vi "RLC Transfer Function Magnitude.vi"(0 "Start frequency, Hz":dbl, 1 "Circuit Type":T2, 5 "Stop frequency, Hz":dbl=10000.0, 7 "Step frequency, Hz":dbl=1.0 format="%#_13g", 11 "error in (no error)":errorcluster, 12 "R, Ohm":dbl=10.0 format="%#_13g", 13 "L, H":dbl=0.01 format="%#_13g", 14 "C, F":dbl=7.5e-06 format="%#_13g") -> (4 "RLC Circuit Transfer function (magnitude)":cluster{"X":dbl[], "Y":dbl[]}(graph), 6 "RLC Circuit Transfer function\n (magnitude) Image Data":T1, 8 "RLC Circuit Transfer function (magnitude) Picture":picture, 10 "JSON string":string, 15 "error out":errorcluster)   [LabVIEW 2019]
uses:
  Types/Circuit Type Enum.ctl
  <vilib>/picture/picture.llb/imagedata.ctl
  XY Graph Data Type.ctl
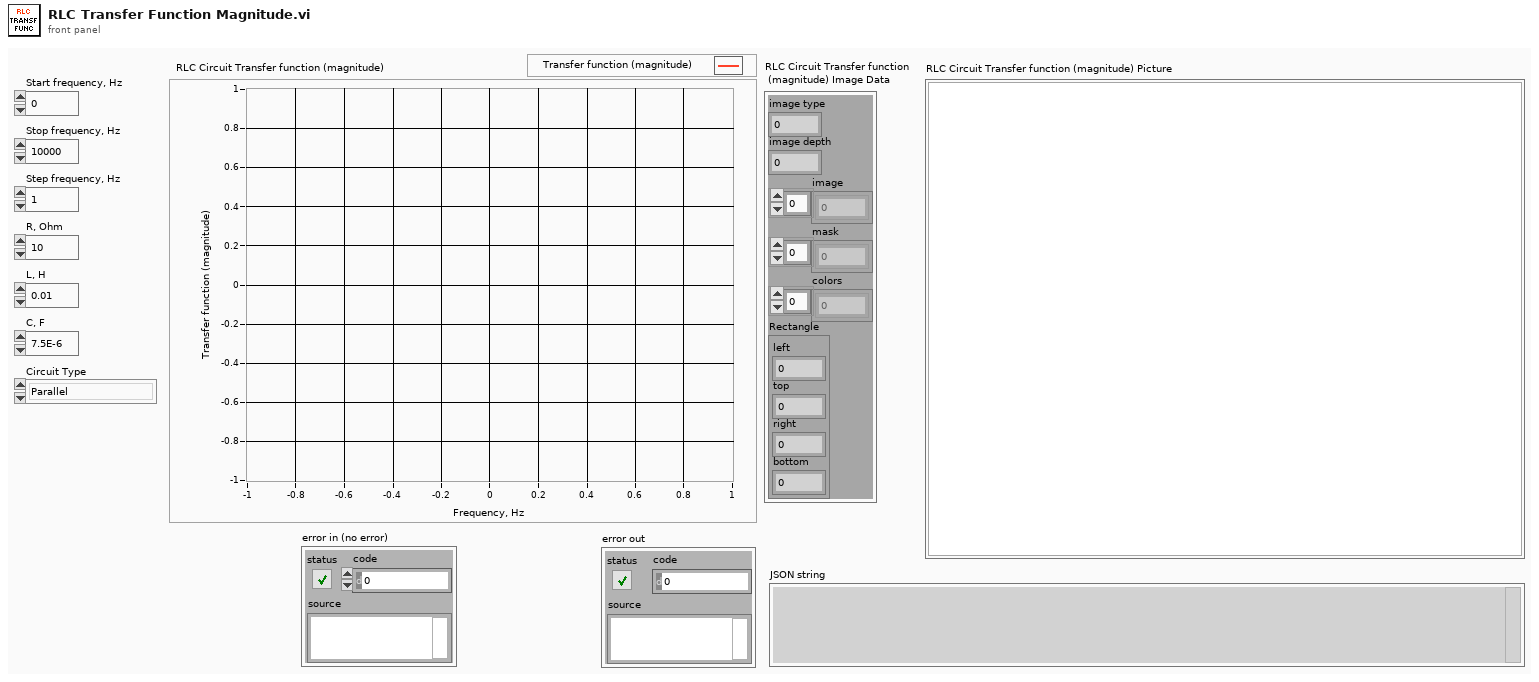
[diagram p1: front panel]
types:
  T1 = typedef "imagedata.ctl" = cluster{"image type":i32, "image depth":i32, "image":u8[], "mask":u8[], "colors":u32[], "Rectangle":cluster{"left":i16, "top":i16, "right":i16, "bottom":i16}}
  T2 = typedef "Circuit Type Enum.ctl" = enum16{"Parallel", "Serial"}
  T3 = typedef "XY Graph Data Type.ctl" = cluster{"X":dbl[], "Y":dbl[]}
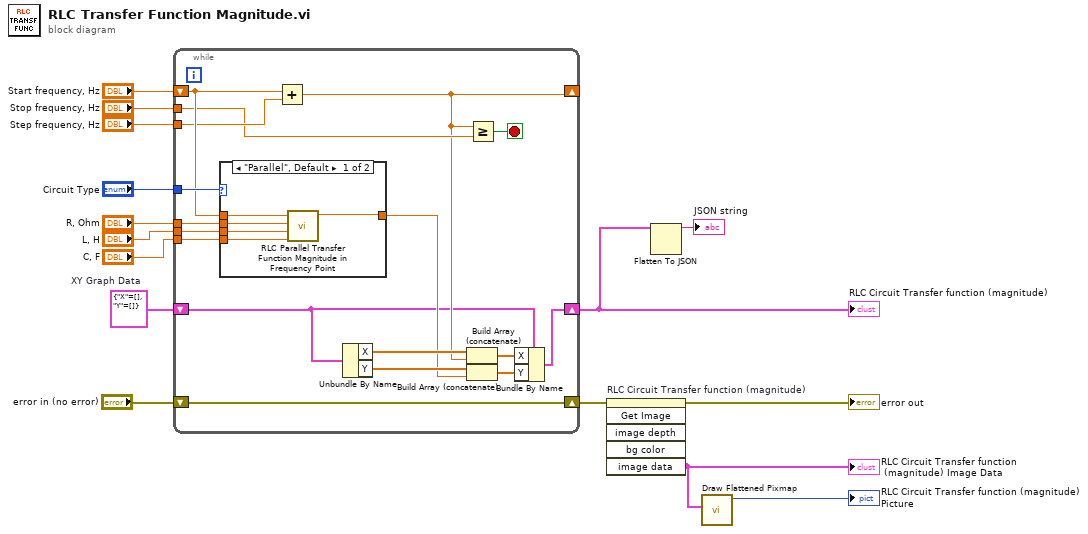
[diagram p0: block diagram]
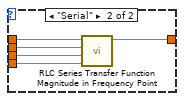
[diagram p2: hidden frame]
diagram:
  w3 = T3 {"X"=[], "Y"=[]}  # XY Graph Data
  n1 = while {
    tunnel: "R, Ohm" -> [w32]
    tunnel: "L, H" -> [w31]
    tunnel: "C, F" -> [w30]
    tunnel: "Circuit Type" -> [w29]
    tunnel: "Stop frequency, Hz" -> [w25]
    tunnel: "Step frequency, Hz" -> [w27]
    shift-right: [w21] -> _
    shift-left: "Start frequency, Hz" -> [w28]
    shift-right: [w16] -> w2
    shift-left: w3 -> [w19]
    shift-right: [w24] -> w7
    shift-left: "error in (no error)" -> [w24]
    stop <- w26 stop-if-true
    n2 = case shown="\"Parallel\", Default" w29 {
      tunnel: w32 -> [w36 w42]
      tunnel: w31 -> [w35 w41]
      tunnel: w30 -> [w34 w40]
      tunnel: w28 -> [w37 w39]
      tunnel: [w33 w38] -> w20
      frame "Parallel", Default {
        n3 = call "RLC Parallel Transfer Function Magnitude in Frequency Point.vi"("C, F"=w34, "L, H"=w35, "R, Ohm"=w36, "F, Hz"=w37) -> ("H(f)"=w33:dbl)  [unwired: 7 in]
      }
      frame "Serial" {
        n4 = call "RLC Series Transfer Function Magnitude in Frequency Point.vi"("C, F"=w40, "L, H"=w41, "R, Ohm"=w42, "F, Hz"=w39) -> ("H(f)"=w38:dbl)  [unwired: 7 in]
      }
    }
    n5 = Add(x=w28, y=w27) -> (x+y=w21:dbl)
    n6 = Unbundle By Name(w19) -> ("X"=w23:dbl[], "Y"=w22:dbl[])
    n7 = Build Array (concatenate)(w23, w21) -> (w18:dbl[])
    n8 = Build Array (concatenate)(w22, w20) -> (w17:dbl[])
    n9 = Greater Or Equal?(x=w21, y=w25) -> (x >= y?=w26:bool)
    n10 = Bundle By Name(cluster=w19, "X"=w18, "Y"=w17) -> (w16:T3)
  }
  "RLC Circuit Transfer function (magnitude)" <- w2
  n11 = invoke on="RLC Circuit Transfer function (magnitude)" class="XYGraph (strict)" method="Get Image"(error in=w7) -> (error out=→"error out":errorcluster, "image data"=w4:T1)  [unwired: 5 in, 4 out]
  "RLC Circuit Transfer function\n (magnitude) Image Data" <- w4
  n12 = Flatten To JSON(anything=w2) -> (JSON string=→"JSON string":string)  [unwired: 2 in, 1 out]
  n13 = call <vilib>:"Draw Flattened Pixmap.vi"("image data"=w4) -> ("new picture"=→"RLC Circuit Transfer function (magnitude) Picture":picture)  [unwired: 8 in]
